vi "Set__slk_mt.vi"(7 "values":string[][](array[string]), 8 "error in (no error)":errorcluster, 11 "boolean in":refnum<class "Boolean__slk_mt.lvclass">) -> (0 "error out":errorcluster, 3 "boolean out":refnum<class "Boolean__slk_mt.lvclass">)   [LabVIEW 2010, in "Lazyboots Menu Tool.lvlib" / "Boolean__slk_mt.lvclass"]
doc: "Sets the values to the control on GUI.\n\n<b>Values:</b>\n[ [Section, Key, Value], [Section, Key, Value], ..., [Section, Key, Value] ]"
uses:
  Boolean__slk_mt.lvclass
  Boolean__slk_mt.lvclass/Boolean__slk_mt.ctl
panel:
  # "Set__slk_mt.vi\nSets the values to the control on GUI.\n\nNOTICE -- YOU MUST LEAVE THIS NOTICE IN PLACE.\n\nCopyright (c) 2011, LIANG LIU Shawn.Liu.cn@gmail.com\nAll rights reserved.\n\nRedistribution and use in source and binary forms, with or without modification, are permitted provided that the following conditions are met:\n-Redistributions of source code must retain the above copyright notice, this list of conditions and the following disclaimer.\n-Redistributions in binary form must reproduce the above copyright notice, this list of conditions and the following disclaimer in the documentation and/or other materials provided with the distribution.\n-Neither the name of the eLp nor the names of its contributors may be used to endorse or promote products derived from this software without specific prior written permission.\n\nTHIS SOFTWARE IS PROVIDED BY THE COPYRIGHT HOLDERS AND CONTRIBUTORS \"AS IS\" AND ANY EXPRESS OR IMPLIED WARRANTIES, INCLUDING, BUT NOT LIMITED TO, THE IMPLIED WARRANTIES OF MERCHANTABILITY AND FITNESS FOR A PARTICULAR PURPOSE ARE DISCLAIMED. IN NO EVENT SHALL THE COPYRIGHT HOLDER OR CONTRIBUTORS BE LIABLE FOR ANY DIRECT, INDIRECT, INCIDENTAL, SPECIAL, EXEMPLARY, OR CONSEQUENTIAL DAMAGES (INCLUDING, BUT NOT LIMITED TO, PROCUREMENT OF SUBSTITUTE GOODS OR SERVICES; LOSS OF USE, DATA, OR PROFITS; OR BUSINESS INTERRUPTION) HOWEVER CAUSED AND ON ANY THEORY OF LIABILITY, WHETHER IN CONTRACT, STRICT LIABILITY, OR TORT (INCLUDING NEGLIGENCE OR OTHERWISE) ARISING IN ANY WAY OUT OF THE USE OF THIS SOFTWARE, EVEN IF ADVISED OF THE POSSIBILITY OF SUCH DAMAGE."
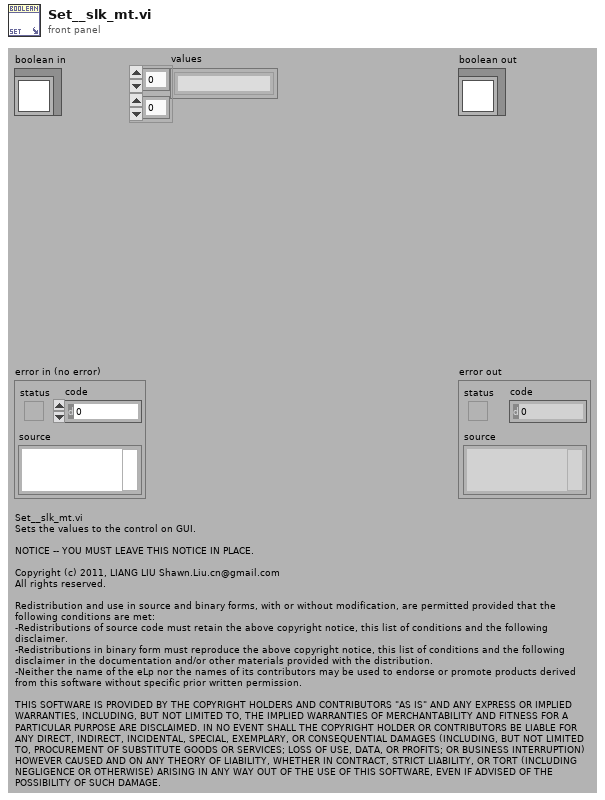
[diagram p1: front panel]
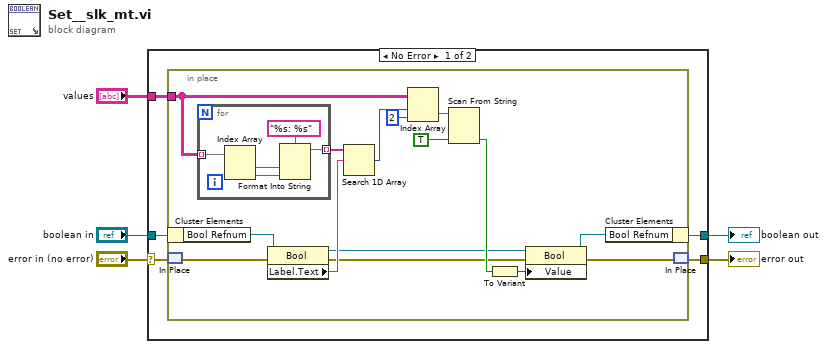
[diagram p0: block diagram]
diagram:
  n1 = case shown="No Error" "error in (no error)" {
    selector: "error in (no error)" -> [w8 w32]
    tunnel: "values" -> [w10 _]
    tunnel: "boolean in" -> [w9 w31]
    tunnel: [w7 w32] -> w2
    tunnel: [w6 w31] -> w1
    frame No Error {
      n2 = in-place {
        in-place-border: w10 -> [w21]
        n3 = in-place-cluster #1(w9) -> ("Bool Refnum"=w13:refnum<vi>)
        n4 = in-place-match #2(w8) -> (w11:errorcluster)
        n5 = for {
          tunnel: w21 -> [w30] mode=indexing
          tunnel: [w26] -> w25 mode=indexing
          n6 = Index Array(array=w30) -> (element #1=w28:string, element #2=w27:string)  [unwired: 2 in]
          n7 = Format Into String(format string="%s: %s", w28, w27) -> (resulting string=w26:string)  [unwired: 2 in, 1 out]
        }
        n8 = property class="Bool"(reference=w13, error in=w11) -> (reference out=w15:refnum<vi>, error out=w16:errorcluster, "Label.Text"=w22:string)
        n9 = Search 1D Array(1D array=w25, element=w22) -> (index of element=w23:i32)  [unwired: 1 in]
        n10 = Index Array(array=w21, index (row)=w23, index (col)=2 ("disabled index (col)")) -> (element=w18:string)
        n11 = Scan From String(input string=w18, default 1=TRUE) -> (output 1=w19:bool)  [unwired: 3 in, 3 out]
        n12 = To Variant(anything=w19) -> (Variant=w17:variant)
        n13 = property class="Bool"(reference=w15, error in=w16, "Value"=w17) -> (reference out=w14:refnum<vi>, error out=w12:errorcluster)
        n14 = in-place-cluster #1("Bool Refnum"=w14) -> (w6:refnum<class "Boolean__slk_mt.lvclass">)
        n15 = in-place-match #2(w12) -> (w7:errorcluster)
      }
    }
    frame Error {
    }
  }
  "error out" <- w2
  "boolean out" <- w1
